vi "Get SLSC Switch Description.vi"(8 "error in (no error)":errorcluster, 11 "SLSC Switch Custom Device Ref in":T1 format="%.0x") -> (0 "error out":errorcluster, 2 "Description":string, 3 "SLSC Switch Custom Device Ref out":T1 format="%.0x")   [LabVIEW 2017, in "SLSC Switch Scripting.lvlib"]
uses:
  SLSC Switch Scripting.lvlib
  <vilib>/NI Veristand/Custom Device API/Custom Device Item Ref.ctl
  <vilib>/NI VeriStand/Custom Device API/Custom Device API.lvlib
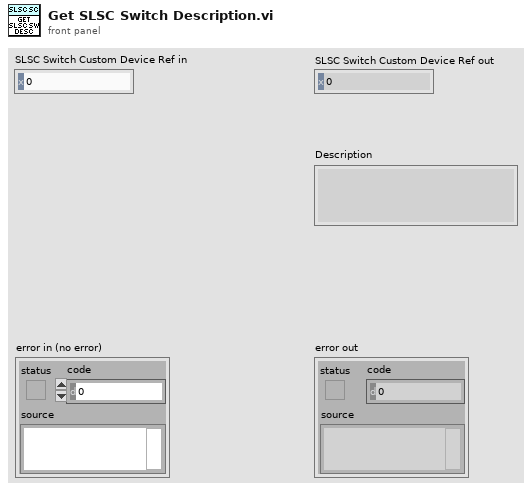
[diagram p1: front panel]
types:
  T1 = typedef "Custom Device API.lvlib/Custom Device Item Ref.ctl" = u64
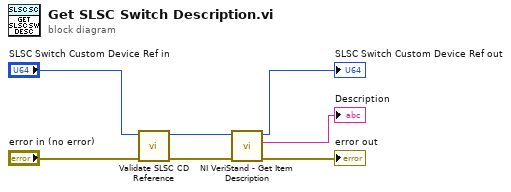
[diagram p0: block diagram]
diagram:
  n1 = call "Validate SLSC CD Reference.vi"("error in (no error)"="error in (no error)", "SLSC Switch Custom Device Ref in"="SLSC Switch Custom Device Ref in") -> ("error out"=w3:errorcluster, "SLSC Switch Custom Device Ref out"=w1:T1)  [unwired: 8 in]
  n2 = call <vilib>:"NI VeriStand - Get Item Description.vi"("error in (no error)"=w3, "Item Ref in"=w1) -> ("error out"=→"error out":errorcluster, "Description"=→"Description":string, "Item Ref out"=→"SLSC Switch Custom Device Ref out":T1)  [unwired: 6 in, 1 out]
